vi "Keyence LJ-V7000 Read Profiles(for High-Speed Data Communication).vi"() -> ()   [LabVIEW 2014]
doc: "This example mainly indicates how to acquire profiles from controllers by using <B>Read Profiles (for High-Speed Communication)</B> VI via high-speed communication. \n\n<B>Note</B>:\nIf you execute this example, set the operation mode of the controller to the high-speed mode."
uses:
  Public/constant/Comm Interface.ctl
  Public/Clusters/Ethernet Config.ctl
  Public/Clusters/High-Speed Comm Start Req.ctl
  Public/constant/High-Speed Comm Start Pos.ctl
  Public/constant/High-Speed Receive Ratio.ctl
  Public/Clusters/Profile Info.ctl
  State Machine State2.ctl
  Keyence LJ-V7000.lvlib
panel:
  out "Timeout Cnt":u32
  out "Height Image":dbl[][](graph)
  out "Read Cnt":u32
  out "Notify":u32
  out "Buf Usage Rate":u32
  out "Profile Info":T1
  in  "Start Req":T2={"High-Speed Comm Start Pos"=2, "Read Profile Cnt"=100, "High-Speed Receive Ratio"=16} {"High-Speed Receive Ratio" items=["LOWEST"=0, "LOW"=16, "MIDDLE"=17, "HIGH"=18, "HIGHEST"=32]; "High-Speed Comm Start Pos" items=["SEND COMPLETE POS", "OLDEST", "NEXT"]}
  in  "Port No":u16
  in  "Stop Monitoring":bool
  in  "Start Monitoring":bool
  in  "Stop High Speed Comm":bool
  in  "Start High Speed Comm":bool
  in  "Stop VI":bool
  in  "Ethernet Config":T5={"IP Address"=[192, 168, 0, 1], "Port No"=24691}
  in  "Comm Interface":T6
  # "High Speed Data Communication Start/Stop"
  # "Read Profiles Start/Stop"
  # "Communication Configuration"
  # "Output from Read Profiles VI"
  # "Communication Configuration\nfor High Speed Communication"
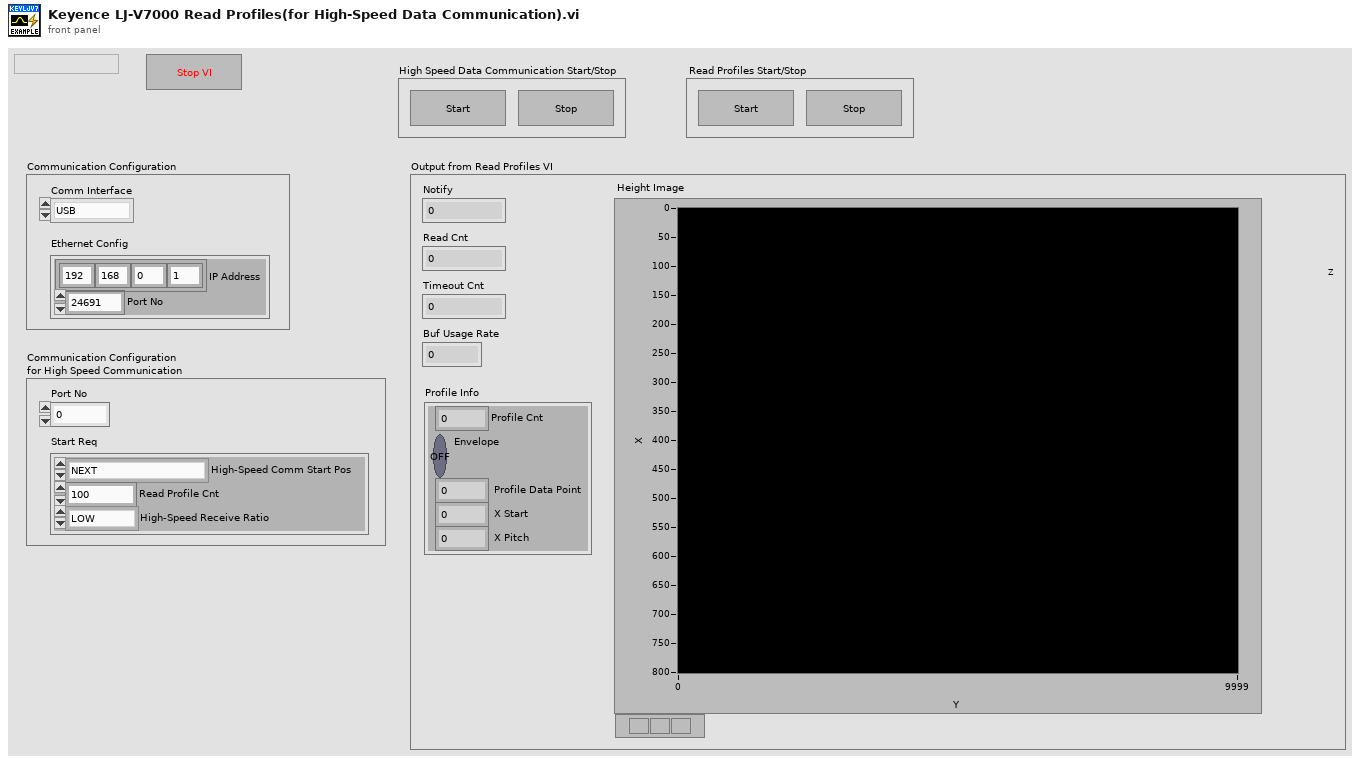
[diagram p1: front panel]
types:
  T1 = typedef "Keyence LJ-V7000.lvlib/Profile Info.ctl" = cluster{"Profile Cnt":u8, "Envelope":bool, " Profile Data Point":u16, " X Start":i32, " X Pitch":i32}
  T2 = typedef "Keyence LJ-V7000.lvlib/High-Speed Comm Start Req.ctl" = cluster{"High-Speed Comm Start Pos":T3, "Read Profile Cnt":u32, "High-Speed Receive Ratio":T4}
  T3 = typedef "Keyence LJ-V7000.lvlib/High-Speed Comm Start Pos.ctl" = u8
  T4 = typedef "Keyence LJ-V7000.lvlib/High-Speed Receive Ratio.ctl" = u8
  T5 = typedef "Keyence LJ-V7000.lvlib/Ethernet Config.ctl" = cluster{"IP Address":u8[], "Port No":u16}
  T6 = typedef "Keyence LJ-V7000.lvlib/Comm Interface.ctl" = enum8{"USB", "ETHERNET"}
  T7 = typedef "State Machine State2.ctl" = enum16{"Idle", "Start High Speed Comm", "Stop High Speed Comm", "Start Monitoring", "Stop Monitoring"}
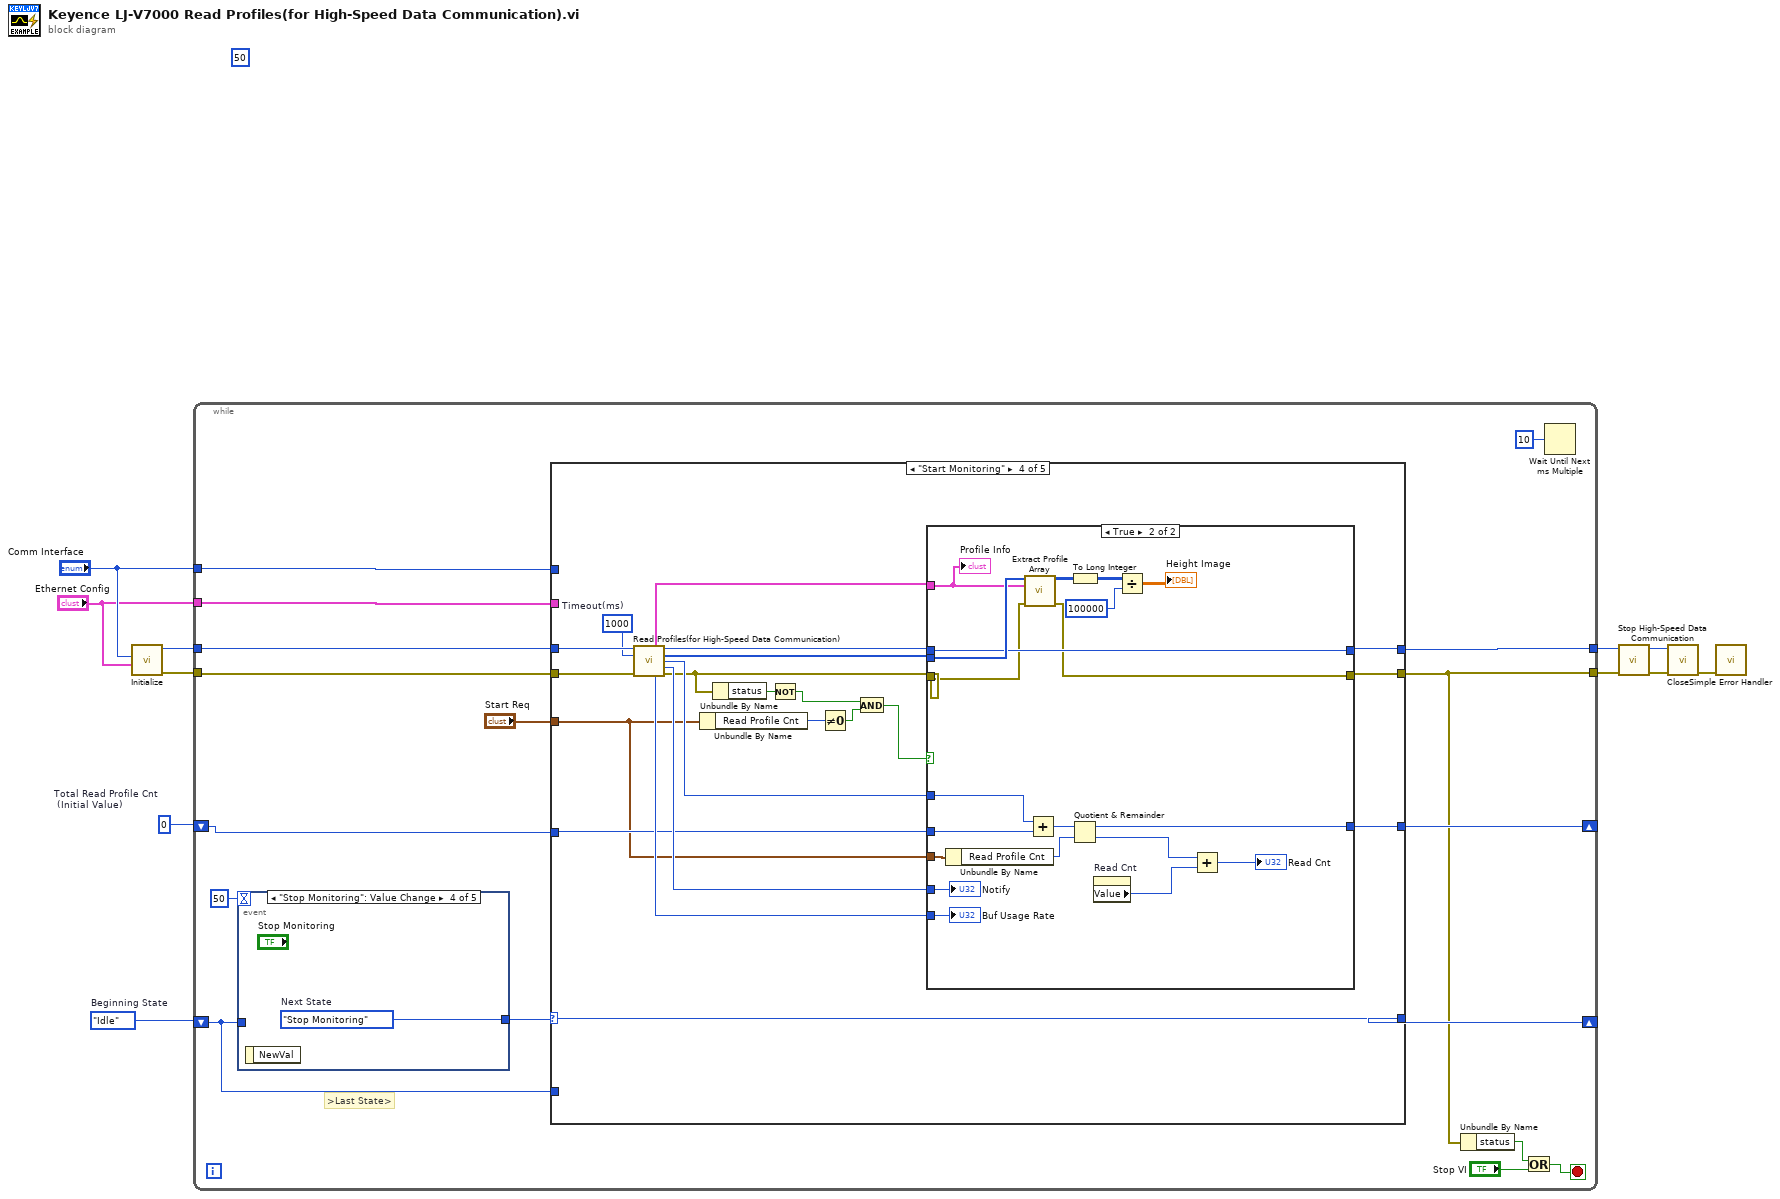
[diagram p0: block diagram]
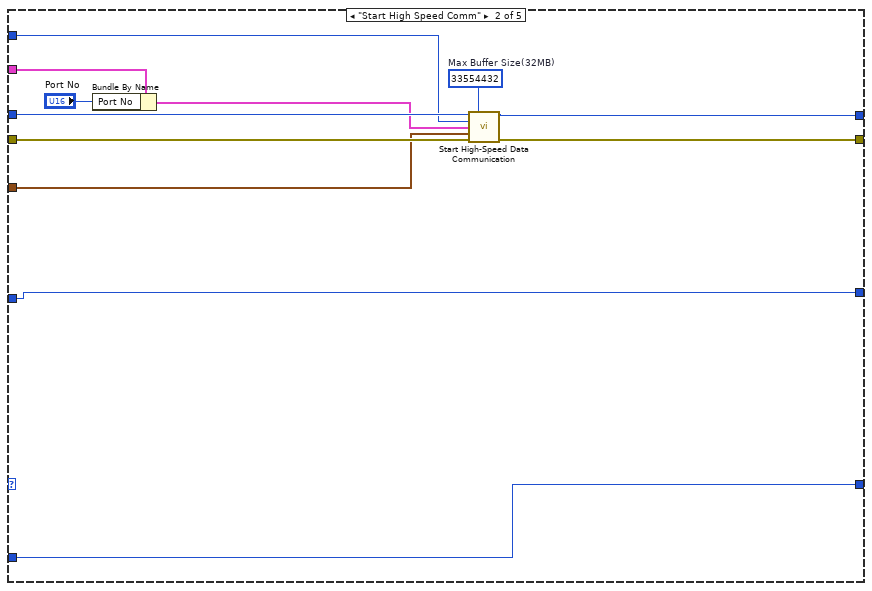
[diagram p3: hidden frame]
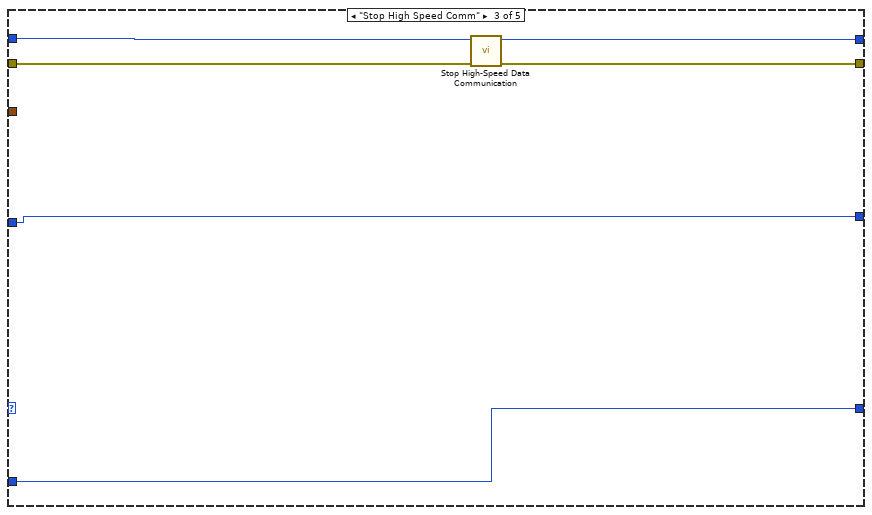
[diagram p4: hidden frame]
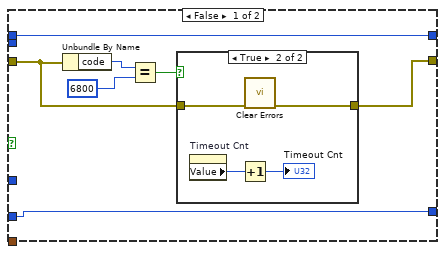
[diagram p5: hidden frame]
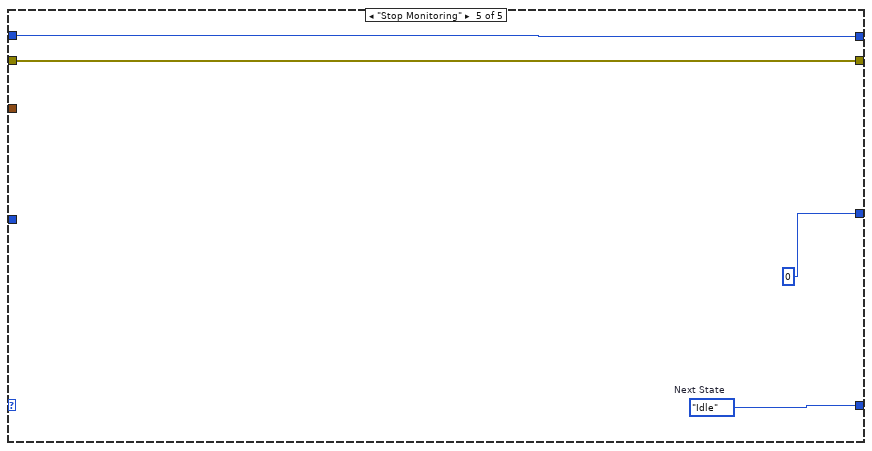
[diagram p7: hidden frame]
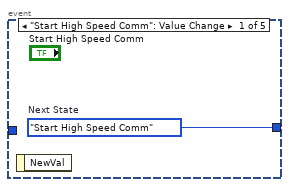
[diagram p8: hidden frame]
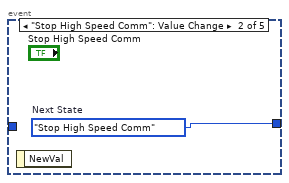
[diagram p9: hidden frame]
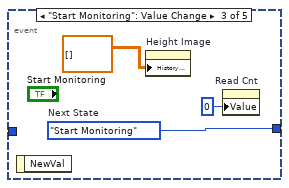
[diagram p10: hidden frame]
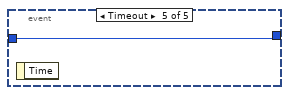
[diagram p11: hidden frame]
diagram:
  w5 = u32 0  # Total Read Profile Cnt  (Initial Value)
  w8 = State_Machine_State2."Idle"  # Beginning State
  (unwired) 50
  n1 = call "Initialize.vi"("Ethernet Config"="Ethernet Config", "Comm Interface"="Comm Interface") -> ("error out"=w11:errorcluster, "Device ID out"=w10:i32)  [unwired: 8 in]
  n2 = while {
    shift-right: [w18] -> _
    shift-left: w8 -> [w17]
    tunnel: w11 -> [w23]
    tunnel: w10 -> [w22]
    tunnel: [w13] -> w2
    tunnel: [w19] -> w1
    tunnel: "Comm Interface" -> [w21]
    tunnel: "Ethernet Config" -> [w20]
    shift-right: [w16] -> _
    shift-left: w5 -> [w15]
    stop <- w26 stop-if-true
    # ">Last State>"
    n3 = event shown="[3] \"Stop Monitoring\": Value Change" {
      selector: _ -> [_ _ _ _ _]
      dyn-events: _ -> [_ _ _ _ _]
      timeout: 50 -> [_ _ _ _ _]
      tunnel: w17 -> [_ _ _ _ w114]
      tunnel: [w108 w109 w112 w113 w114] -> w24
      event "Start High Speed Comm": Value Change {
        w108 = State_Machine_State2."Start High Speed Comm"  # Next State
        n4 = event-data() -> ()  [unwired: 1 in, 1 out]
      }
      event "Stop High Speed Comm": Value Change {
        w109 = State_Machine_State2."Stop High Speed Comm"  # Next State
        n5 = event-data() -> ()  [unwired: 1 in, 1 out]
      }
      event "Start Monitoring": Value Change {
        w112 = State_Machine_State2."Start Monitoring"  # Next State
        n6 = event-data() -> ()  [unwired: 1 in, 1 out]
        n7 = property on="Height Image" class="IntChart (strict)"("History Data"=dbl[][] [] ("履歴データ")) -> ()  [unwired: 2 in, 2 out]
        n8 = property on="Read Cnt" class="DigNum (strict)"("Value"=u32 0 ("Read Cnt")) -> ()  [unwired: 2 in, 2 out]
      }
      event "Stop Monitoring": Value Change {
        w113 = State_Machine_State2."Stop Monitoring"  # Next State
        n9 = event-data() -> ()  [unwired: 1 in, 1 out]
      }
      event Timeout {
        n10 = event-data() -> ()  [unwired: 1 in, 1 out]
      }
    }
    n11 = case shown="\"Start Monitoring\"" w24 {
      selector: w24 -> [w32 _ _ w68 _]
      tunnel: w23 -> [w29 w44 w49 w71 w106]
      tunnel: w22 -> [w30 w43 w48 w70 w107]
      tunnel: w21 -> [_ w42 _ _ _]
      tunnel: w20 -> [_ w41 _ _ _]
      tunnel: [w29 w38 w50 w63 w106] -> w13
      tunnel: [w30 w37 w47 w58 w107] -> w19
      tunnel: [w32 w35 w46 w68 w105] -> w18
      tunnel: w17 -> [_ w35 w46 _ _]
      tunnel: [w31 w34 w45 w60 u32 0] -> w16
      tunnel: w15 -> [w31 w34 w45 w64 _]
      tunnel: "Start Req" -> [_ w33 _ w56 _]
      frame "Idle", Default {
      }
      frame "Start High Speed Comm" {
        w36 = u32 33554432  # Max Buffer Size(32MB)
        n12 = Bundle By Name(cluster=w41, "Port No"="Port No") -> (w39:T5)
        n13 = call "Start High-Speed Data Communication.vi"("Device ID (0)"=w43, "Max Buffer Size"=w36, "Comm Interface"=w42, "Ethernet Config"=w39, "Start Req"=w33, "error in (no error)"=w44) -> ("Device ID out"=w37:i32, "error out"=w38:errorcluster)  [unwired: 8 in]
      }
      frame "Stop High Speed Comm" {
        n14 = call "Stop High-Speed Data Communication.vi"("error in (no error)"=w49, "Device ID (0)"=w48) -> ("error out"=w50:errorcluster, "Device ID out"=w47:i32)  [unwired: 8 in]
      }
      frame "Start Monitoring" {
        w69 = u32 1000  # Timeout(ms)
        n15 = call "Read Profiles(for High-Speed Data Communication).vi"("Device ID (0)"=w70, "Timeout"=w69, "error in (no error)"=w71) -> ("Profile Info"=w62:T1, "Device ID out"=w59:i32, "Profile Data"=w61:u32[], "Rsp Profile Cnt"=w65:u32, "Notify"=w66:u32, "Buf Usage Rate"=w67:u32, "error out"=w57:errorcluster)  [unwired: 6 in]
        n16 = Unbundle By Name(w56) -> ("Read Profile Cnt"=w55:u32)
        n17 = Unbundle By Name(w57) -> ("status"=w54:bool)
        n18 = Not(x=w54) -> (.not. x?=w52:bool)
        n19 = Not Equal To 0?(x=w55) -> (x != 0?=w53:bool)
        n20 = And(x=w52, y=w53) -> (x .and. y?=w51:bool)
        n21 = case shown="True" w51 {
          tunnel: w67 -> [_ w103]
          tunnel: w66 -> [_ w102]
          tunnel: w65 -> [_ w101]
          tunnel: w64 -> [w72 w100]
          tunnel: [w75 w85] -> w63
          tunnel: w62 -> [_ w87]
          tunnel: w61 -> [_ w99]
          tunnel: w57 -> [w74 w84]
          tunnel: w56 -> [_ w94]
          tunnel: [w72 w90] -> w60
          tunnel: w59 -> [w73 w86]
          tunnel: [w73 w86] -> w58
          frame False {
            n22 = Unbundle By Name(w74) -> ("code"=w78:i32)
            n23 = Equal?(x=w78, y=6800) -> (x = y?=w76:bool)
            n24 = case shown="True" w76 {
              tunnel: w74 -> [w79 w83]
              tunnel: [w79 w82] -> w75
              frame False {
              }
              frame True {
                n25 = property on="Timeout Cnt" class="DigNum (strict)"() -> ("Value"=w80:u32)  [unwired: 2 in, 2 out]
                n26 = Increment(x=w80) -> (x+1=→"Timeout Cnt":u32)
                n27 = call <vilib>:"Clear Errors.vi"("error in (no error)"=w83) -> ("error out"=w82:errorcluster)  [unwired: 5 in, 1 out]
              }
            }
          }
          frame True {
            n28 = Unbundle By Name(w94) -> ("Read Profile Cnt"=w92:u32)
            n29 = call "Extract Profile Array.vi"("Profile Data"=w99, "Profile Info"=w87, "error in (no error)"=w84) -> ("Profile A Array1"=w96:u32[][], "error out"=w85:errorcluster)  [unwired: 8 in, 3 out]
            n30 = Add(x=w101, y=w100) -> (x+y=w93:u32)
            n31 = To Long Integer(number=w96) -> (32bit integer=w97:i32[][])
            n32 = Quotient & Remainder(x=w93, y=w92) -> (x-y*floor(x/y)=w90:u32, floor(x/y)=w88:u32)
            n33 = property on="Read Cnt" class="DigNum (strict)"() -> ("Value"=w89:u32)  [unwired: 2 in, 2 out]
            n34 = Divide(x=w97, y=100000) -> (x/y=→"Height Image":dbl[][])
            n35 = Add(x=w88, y=w89) -> (x+y=→"Read Cnt":u32)
            "Buf Usage Rate" <- w103
            "Notify" <- w102
            "Profile Info" <- w87
          }
        }
      }
      frame "Stop Monitoring" {
        w105 = State_Machine_State2."Idle"  # Next State
      }
    }
    n36 = Unbundle By Name(w13) -> ("status"=w14:bool)
    n37 = Or(x=w14, y="Stop VI") -> (x .or. y?=w26:bool)
    n38 = Wait Until Next ms Multiple(millisecond multiple=u32 10 ("ミリ秒倍数")) -> ()  [unwired: 1 out]
  }
  n39 = call "Stop High-Speed Data Communication.vi"("error in (no error)"=w2, "Device ID (0)"=w1) -> ("error out"=w3:errorcluster, "Device ID out"=w4:i32)  [unwired: 8 in]
  n40 = call "Close.vi"("error in (no error)"=w3, "Device ID (0)"=w4) -> ("error out"=w9:errorcluster)  [unwired: 8 in, 1 out]
  n41 = call <vilib>:"Simple Error Handler.vi"("error in (no error)"=w9) -> ()  [unwired: 4 in, 5 out]
